vi "Read Config from File.vi"(6 "Comment out unparsable lines":bool=TRUE, 7 "Template (JSON Object)":string="{}", 8 "error in (no error)":errorcluster, 10 "config file path":path) -> (0 "error out":errorcluster, 1 "Template Used (file missing or corrupted)":bool, 2 "<JSON>Config":string, 3 "Config File":refnum<class "JSONConfigFile.lvclass">)   [LabVIEW 2021, in "json.facade.lvlib" / "JSONConfigFile.lvclass"]
doc: "Read in the Configuration from the specified file. If the file does not exists, a supplied Template will be used (if input). The Template should be a JSON Object and may include Comments."
uses:
  JSONConfigFile.lvclass
  JSONConfigFile.lvclass/JSONConfigFile.ctl
  jsontext/Config Files/Config File.lvclass
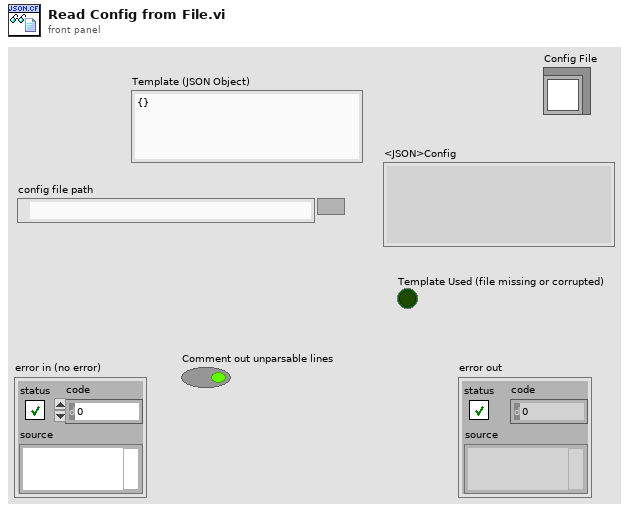
[diagram p1: front panel]
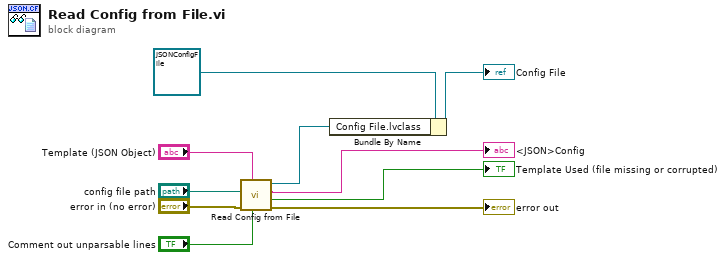
[diagram p0: block diagram]
diagram:
  n1 = call "Read Config from File.vi"("Comment out unparsable lines"="Comment out unparsable lines", "Template (JSON Object)"="Template (JSON Object)", "error in (no error)"="error in (no error)", "config file path"="config file path") -> ("error out"=→"error out":errorcluster, "Template Used (file missing or corrupted)"=→"Template Used (file missing or corrupted)":bool, "<JSON>Config"=→"<JSON>Config":string, "Config File"=w2:refnum<class "Config File.lvclass">)  [unwired: 4 in]
  n2 = Bundle By Name(cluster=refnum<class "JSONConfigFile.lvclass"> refnum ("jsontext.facade.lvlib:Config File.lvclass"), "Config File.lvclass"=w2) -> (→"Config File":refnum<class "JSONConfigFile.lvclass">)
